vi "Add String to Array Elements.vi"(9 "Append String":string, 10 "String Array In":string[](array[string]), 11 "Prepend String":string) -> (2 "String Array Out":string[](array[string]))   [LabVIEW 2016, in "UserInterface.lvlib" / "UserInterface.lvclass"]
doc: "Add a string to each element of an array, either at the start, end of both start and end of each element."
uses:
  UserInterface.lvclass
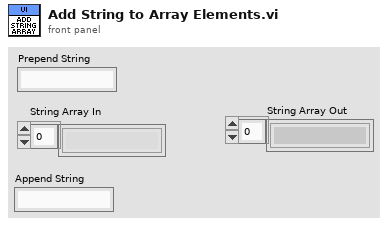
[diagram p1: front panel]
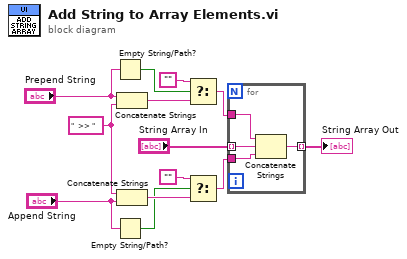
[diagram p0: block diagram]
diagram:
  w3 = "  >> " ("string")
  n1 = Empty String/Path?(string/path="Prepend String") -> (empty?=w11:bool)
  n2 = Empty String/Path?(string/path="Append String") -> (empty?=w4:bool)
  n3 = Concatenate Strings("Prepend String", w3) -> (w8:string)
  n4 = Concatenate Strings(w3, "Append String") -> (w6:string)
  n5 = Select(t="", s=w11, f=w8) -> (s? t:f=w7:string)
  n6 = Select(t="", s=w4, f=w6) -> (s? t:f=w1:string)
  n7 = for {
    tunnel: "String Array In" -> [w17] mode=indexing
    tunnel: [w16] -> w12 mode=indexing
    tunnel: w7 -> [w15]
    tunnel: w1 -> [w14]
    n8 = Concatenate Strings(w15, w17, w14) -> (w16:string)
  }
  "String Array Out" <- w12
